vi "Tracer_Create.vi"(8 "Error In":errorcluster) -> (0 "Error Out":errorcluster)   [LabVIEW 2018, in "TracerLibrary.lvlib" / "Tracer.lvclass"]
uses:
  Tracer.lvclass
  protected/Tracer_ObjectAttributes.ctl
  protected/Tracer_ClassAttributes.vi
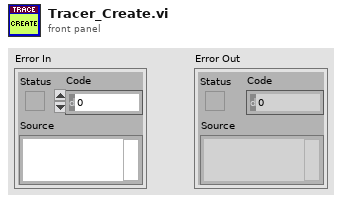
[diagram p1: front panel]
types:
  T1 = typedef "TracerLibrary.lvlib/Tracer.lvclass/Tracer_ObjectAttributes.ctl" = cluster{"TraceContainer":variant}
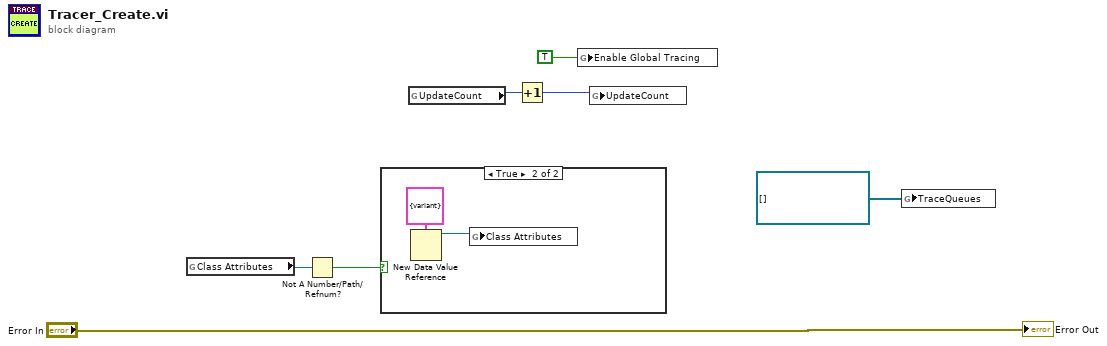
[diagram p0: block diagram]
diagram:
  n1 = global read "Tracer_ClassAttributes.vi" "Class Attributes"() -> (w6:refnum<data-value>)
  n2 = Not A Number/Path/Refnum?(number/path/refnum=w6) -> (NaN/Path/Refnum?=w5:bool)
  n3 = case shown="True" w5 {
    frame False {
    }
    frame True {
      n4 = New Data Value Reference(data value=T1 {"TraceContainer"=variant} ("ObjectAttributes")) -> (data value reference=w8:refnum<data-value>)  [unwired: 1 in, 1 out]
      n5 = global write "Tracer_ClassAttributes.vi" "Class Attributes"(w8) -> ()
    }
  }
  n6 = global read "Tracer_ClassAttributes.vi" "UpdateCount"() -> (w3:i32)
  n7 = Increment(x=w3) -> (x+1=w2:i32)
  n8 = global write "Tracer_ClassAttributes.vi" "Enable Global Tracing"(TRUE ("TRACE Enable")) -> ()
  n9 = global write "Tracer_ClassAttributes.vi" "UpdateCount"(w2) -> ()
  n10 = global write "Tracer_ClassAttributes.vi" "TraceQueues"(refnum<queue>[] [] ("TraceQueues")) -> ()
  "Error Out" <- "Error In"
